vi "Строку в числовые данные мишеней (SubVI).vi"(12 "Строка с числовыми параметрами мишени":string) -> (13 "Остаток строки":string, 23 "Кластер числовых параметров мишеней":T1)   [LabVIEW 2015]
doc: "Преобразование строки с числовыми параметрами мишени в числа - параметры мишеней"
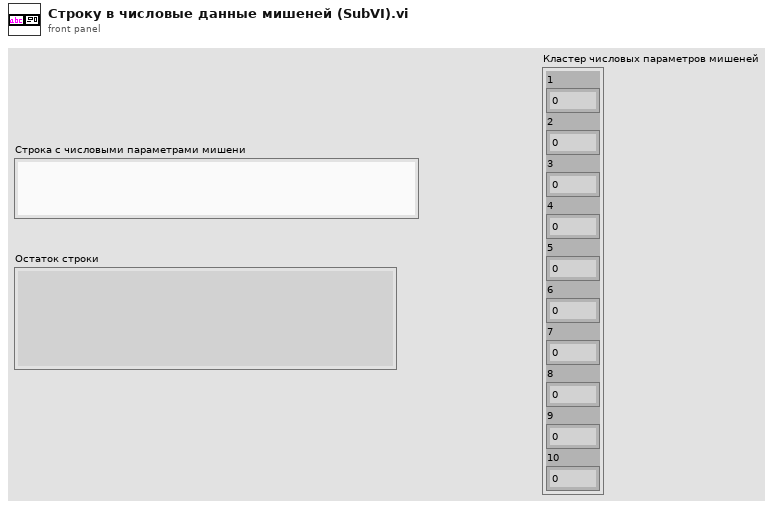
[diagram p1: front panel]
types:
  T1 = cluster{"1":u16, "2":u16, "3":u16, "4":u16, "5":u16, "6":u16, "7":u16, "8":u16, "9":u16, "10":u16}
  T2 = cluster{"default value 1":u16, "default value 1":u16, "default value 1":u16, "default value 1":u16, "default value 1":u16, "default value 1":u16, "default value 1":u16, "default value 1":u16, "default value 1":u16, "default value 1":u16}
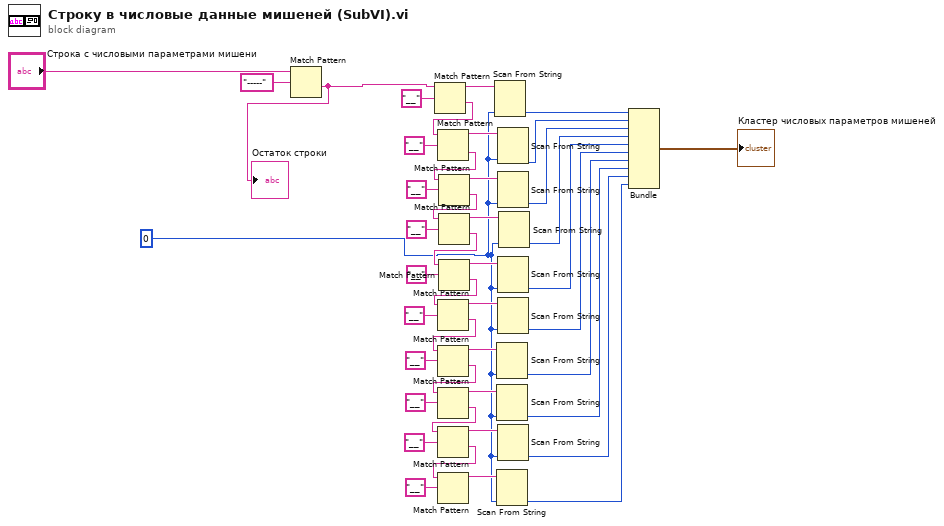
[diagram p0: block diagram]
diagram:
  w1 = u16 0 ("default value 1")
  n1 = Match Pattern(string="Строка с числовыми параметрами мишени", regular expression="-----") -> (after substring=w41:string)  [unwired: 1 in, 3 out]
  "Остаток строки" <- w41
  n2 = Match Pattern(string=w41, regular expression="__" ("delimiter (Tab)")) -> (before substring=w39:string, after substring=w40:string)  [unwired: 1 in, 2 out]
  n3 = Match Pattern(string=w40, regular expression="__" ("delimiter (Tab)")) -> (before substring=w32:string, after substring=w34:string)  [unwired: 1 in, 2 out]
  n4 = Match Pattern(string=w34, regular expression="__" ("delimiter (Tab)")) -> (before substring=w6:string, after substring=w30:string)  [unwired: 1 in, 2 out]
  n5 = Match Pattern(string=w30, regular expression="__" ("delimiter (Tab)")) -> (before substring=w5:string, after substring=w8:string)  [unwired: 1 in, 2 out]
  n6 = Match Pattern(string=w8, regular expression="__" ("delimiter (Tab)")) -> (before substring=w25:string, after substring=w24:string)  [unwired: 1 in, 2 out]
  n7 = Match Pattern(string=w24, regular expression="__" ("delimiter (Tab)")) -> (before substring=w23:string, after substring=w27:string)  [unwired: 1 in, 2 out]
  n8 = Match Pattern(string=w27, regular expression="__" ("delimiter (Tab)")) -> (before substring=w22:string, after substring=w13:string)  [unwired: 1 in, 2 out]
  n9 = Match Pattern(string=w13, regular expression="__" ("delimiter (Tab)")) -> (before substring=w14:string, after substring=w19:string)  [unwired: 1 in, 2 out]
  n10 = Match Pattern(string=w19, regular expression="__" ("delimiter (Tab)")) -> (before substring=w44:string, after substring=w17:string)  [unwired: 1 in, 2 out]
  n11 = Match Pattern(string=w17, regular expression="__" ("delimiter (Tab)")) -> (before substring=w12:string)  [unwired: 1 in, 3 out]
  n12 = Scan From String(input string=w39, default 1=w1) -> (output 1=w42:u16)  [unwired: 3 in, 3 out]
  n13 = Scan From String(input string=w22, default 1=w1) -> (output 1=w20:u16)  [unwired: 3 in, 3 out]
  n14 = Scan From String(input string=w14, default 1=w1) -> (output 1=w11:u16)  [unwired: 3 in, 3 out]
  n15 = Scan From String(input string=w12, default 1=w1) -> (output 1=w9:u16)  [unwired: 3 in, 3 out]
  n16 = Scan From String(input string=w32, default 1=w1) -> (output 1=w35:u16)  [unwired: 3 in, 3 out]
  n17 = Scan From String(input string=w6, default 1=w1) -> (output 1=w4:u16)  [unwired: 3 in, 3 out]
  n18 = Scan From String(input string=w25, default 1=w1) -> (output 1=w29:u16)  [unwired: 3 in, 3 out]
  n19 = Scan From String(input string=w23, default 1=w1) -> (output 1=w21:u16)  [unwired: 3 in, 3 out]
  n20 = Scan From String(input string=w44, default 1=w1) -> (output 1=w10:u16)  [unwired: 3 in, 3 out]
  n21 = Scan From String(input string=w5, default 1=w1) -> (output 1=w3:u16)  [unwired: 3 in, 3 out]
  n22 = Bundle("default value 1"=w42, "default value 1"=w35, "default value 1"=w4, "default value 1"=w3, "default value 1"=w29, "default value 1"=w21, "default value 1"=w20, "default value 1"=w11, "default value 1"=w10, "default value 1"=w9) -> (→"Кластер числовых параметров мишеней":T2)  [unwired: 1 in]
